vi "modbus slave new.vi"() -> ()   [LabVIEW 2016, in "MB SLAVE.lvlib"]
uses:
  MB SLAVE.lvlib
  <vilib>/NI/Modbus Library/Network Protocol/Network Slave/daemon status.ctl
  <vilib>/NI/Modbus Library/Network Protocol/Network Slave/TCP/Connection.ctl
  <vilib>/NI/Modbus Library/API/slave/Modbus Slave.lvclass
  <vilib>/NI/Modbus Library/API/Wrapper/Create TCP Slave.vi
  <vilib>/NI/Modbus Library/API/Wrapper/API Main.lvlib
  <vilib>/ptbypt/NI_PtbyPt.lvlib
  <vilib>/NI/Modbus Library/Network Protocol/Network Slave/Network Slave.lvclass
  <vilib>/NI/Modbus Library/Network Protocol/Network Slave/TCP/TCP Slave.lvclass
panel:
  out "MB引用":refnum<class "Modbus Slave.lvclass">
  out "读取采水泵阀":u16[](array[numeric])
  out "读取数采仪软件版本":u16[](array[numeric])
  in  "写入数据传输软件升级":u16[](array[numeric])
  in  "写入仪器固件":u16[](array[numeric])
  in  "写入系统信息":u16[](array[numeric])
  in  "写入系统版本信息":u16[](array[numeric])
  in  "写入仪器告警信息":u16[](array[numeric])
  in  "写入采配水关键参数":u16[](array[numeric])
  in  "写入校准点信息":u16[](array[numeric])
  in  "写入关键参数":u16[](array[numeric])
  in  "写入各参数测量间隔":u16[](array[numeric])
  out "读取各参数测量间隔":u16[](array[numeric])
  in  "写入试剂余量":u16[](array[numeric])
  out "TCP Connection List":T1[](array[typedef])
  out "TCP Connection Count":u32
  out "Daemon Status":T2
  out "读取关键参数":u16[](array[numeric])
  out "status":bool
  in  "写入系统仪器状态":u16[](array[numeric])
  out "读取反控命令":u16[](array[numeric])
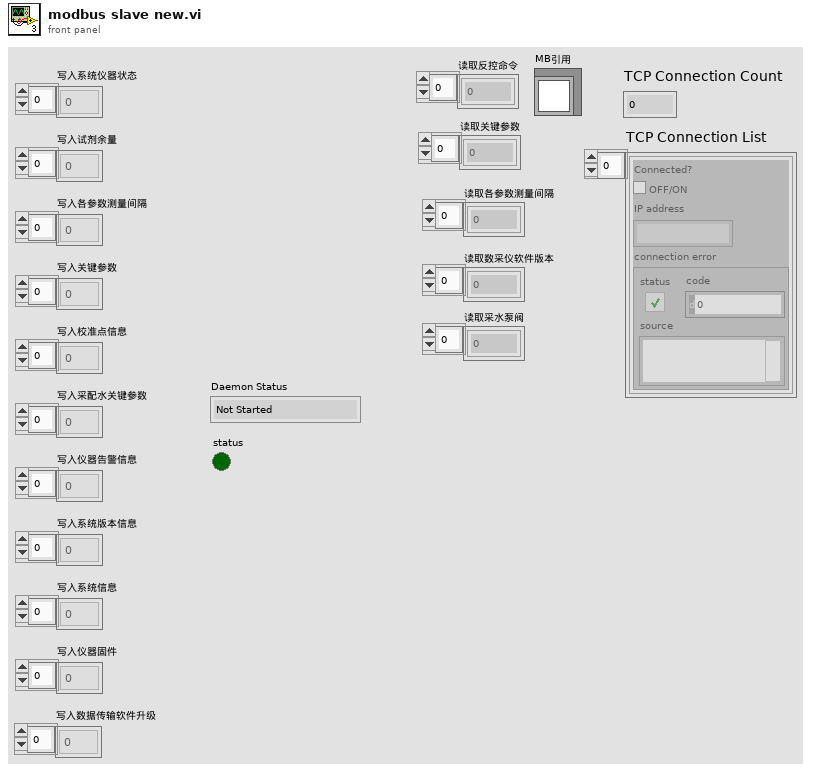
[diagram p1: front panel]
types:
  T1 = typedef "TCP Slave.lvclass/Connection.ctl" = cluster{"Connected?":bool, "IP address":string, "connection error":errorcluster}
  T2 = typedef "Network Slave.lvclass/daemon status.ctl" = enum16{"Not Started", "Running", "Error", "Stopped"}
  T3 = enum16{"", "CODMn", "PH", "氨氮", "总氮", "总磷", "CODCr", "电导率", "水温", "溶解氧", "浊度", "叶绿素", "藻密度", "ORP"}
  T4 = enum16{"i13001", "i13002", "i13003", "i13004", "i13005", "i13006", "i13007", "i13008", "i13009", "i13010", "i13011", "i13012", "i13013", "i13014", "i13015", "i13016", "i13017", "i13101", "i13102", "i13103", "i13104", "i13105", "i13106", "i13107", "i13108", "i13109", "i13110"}
  T5 = cluster{"status":bool, "代码":u16, "source":string}
  T6 = typedef "系统交互.ctl" = cluster{"运行模式":enum16{"维护模式", "常规模式", "应急模式", "质控模式", "性能测试"}, "运行间隔":i16, "流程运行中":bool, "自动运行启动参数":T7, "SYSTEM Interface.总磷总氮类型":enum16{"单模块", "总磷总氮二合一模块", "氨氮总磷二合一模块"}, "多参数运行间隔":i16, "配水时间":dbl, "沉淀时间":dbl, "清洗时间":dbl, "关键参数改变":bool, "温度告警":bool, "湿度告警":bool, "烟感告警":bool, "水浸告警":bool, "开门告警":bool, "SystemTask":enum16{"停机", "待机", "调试", "水样采集", "沉沙", "进样", "仪表测试分析", "反吹", "清洗", "除藻"}, "PumpState":enum16{"--", "只用泵1", "只用泵2", "双泵交替"}, "除藻选择":enum16{"不开除藻", "开除藻"}, "报警信息":enum16{"无报警", "断电报警", "采样管理欠压（源水泵故障）", "进样管路欠压（进样泵/增加泵故障）"}, "软件升级":bool, "固件升级":enum16{"无", "CODMn", "氨氮", "总磷", "总氮", "CODCr"}, "数据传输软件升级":bool, "数采仪软件版本":string}
  T7 = typedef "启动参数.ctl" = cluster{"氨氮":bool, "总磷":bool, "总氮":bool, "多参数":bool, "CODmn":bool, "CODCr":bool, "超标留样":bool}
  T8 = enum16{"停机", "待机", "调试", "水样采集", "沉沙", "进样", "仪表测试分析", "反吹", "清洗", "除藻"}
  T9 = enum16{"无报警", "断电报警", "采样管理欠压（源水泵故障）", "进样管路欠压（进样泵/增加泵故障）"}
  T10 = typedef "多参数交互.ctl" = cluster{"pH":bool, "DO":bool, "Turb":bool, "Cond":bool, "Temp":bool, "叶绿素a启用":bool, "蓝绿藻":bool, "藻密度":bool, "orp":bool}
  T11 = typedef "CODMn交互.ctl" = cluster{"COD浓度（mg/L)":dbl, "水样启动时间":timestamp, "加标回收启动时间":timestamp, "CODMn工作状态":enum16{"空闲", "水样测试", "标样核查", "零点核查", "跨度核查", "空白测试", "平行样测试", "加标回收", "空白校准", "标样校准", "初始化（清洗）"}, "多列列表框":i32, "平台试剂余量百分比":sgl, "关键参数":cluster{"测量量程":dbl, "测量精度":dbl, "测量间隔":dbl, "消解温度":dbl, "消解时长":dbl, "空白校准时间":timestamp, "曲线截距":dbl, "曲线斜率":dbl, "测量检出限":dbl, "测量信号值":dbl, "线性相关系数":dbl, "二次多项式系数":dbl, "标样校准时间":timestamp, "稀释倍数":dbl, "三项式系数":dbl, "空白标定系数":dbl, "量程系数":dbl, "F0/ORPA":dbl, "F1/ORPB":dbl, "F2/ORPK":dbl, "F3":dbl, "F4":dbl, "F5":dbl, "F6":dbl, "F7":dbl, "X0/滴定数":dbl, "量程":dbl}, "关键参数改变":bool, "校准信息":cluster{"低标液1浓度":dbl, "低标液1信号值":dbl, "低标液1启用":u16, "低标液2浓度":dbl, "低标液2信号值":dbl, "低标液2启用":u16, "低标液3浓度":dbl, "低标液3信号值":dbl, "低标液3启用":u16, "低标液4浓度":dbl, "低标液4信号值":dbl, "低标液4启用":u16, "低标液5浓度":dbl, "低标液5信号值":dbl, "低标液5启用":u16, "高标液1浓度":dbl, "高标液1信号值":dbl, "高标液1启用":u16, "高标液2浓度":dbl, "高标液2信号值":dbl, "高标液2启用":u16, "高标液3浓度":dbl, "高标液3信号值":dbl, "高标液3启用":u16, "高标液4浓度":dbl, "高标液4信号值":dbl, "高标液4启用":u16, "高标液5浓度":dbl, "高标液5信号值":dbl, "高标液5启用":u16, "低斜率":dbl, "低截距":dbl, "低二次多项式系数":dbl, "低线性相关系数":dbl, "高斜率":dbl, "高截距":dbl, "高二次多项式系数":dbl, "高线性相关系数":dbl}, "校准信息改变":bool, "固件版本号":string, "CODMn模块版本":T12, "协议":u16, "状态告警区":cluster{"系统时间":timestamp, "工作状态":u16, "测量模式":enum16{"待机", "连续模式", "周期模式", "定点模式", "受控模式", "手动模式"}, "告警代码":u16, "故障代码":u16, "日志代码":u16, "软件版本":u16, "F0":sgl, "F1":sgl, "F2":sgl, "F3":sgl, "T":sgl, "H":sgl, "id":u16, "flowid":u16, "量程":u16, "总磷控温温度1":sgl, "营养盐控温温度2":sgl, "ADC":sgl}, "标样核查标液浓度":dbl, "测量数据区":cluster{"空白数据时间":timestamp, "空白实测值":sgl, "标样数据时间":timestamp, "标样实测值":sgl}}
  T12 = typedef "CODMn模块版本.ctl" = enum16{"PLC版", "单片机版", "通用流路版本"}
  T13 = typedef "CODCr交互.ctl" = cluster{"状态告警区":cluster{"系统时间":timestamp, "工作状态":u16, "测量模式":enum16{"待机", "连续模式", "周期模式", "定点模式", "受控模式", "手动模式"}, "告警代码":u16, "故障代码":u16, "日志代码":u16, "软件版本":u16, "F0":sgl, "F1":sgl, "F2":sgl, "F3":sgl, "T":sgl, "H":sgl, "id":u16, "flowid":u16, "量程":u16, "总磷控温温度1":sgl, "营养盐控温温度2":sgl, "ADC":sgl}, "平台试剂余量百分比":sgl, "关键参数":cluster{"测量量程":dbl, "测量精度":dbl, "测量间隔":dbl, "消解温度":dbl, "消解时长":dbl, "空白校准时间":timestamp, "曲线截距":dbl, "曲线斜率":dbl, "测量检出限":dbl, "测量信号值":dbl, "线性相关系数":dbl, "二次多项式系数":dbl, "标样校准时间":timestamp, "稀释倍数":dbl, "三项式系数":dbl, "空白标定系数":dbl, "量程系数":dbl, "F0/ORPA":dbl, "F1/ORPB":dbl, "F2/ORPK":dbl, "F3":dbl, "F4":dbl, "F5":dbl, "F6":dbl, "F7":dbl, "X0/滴定数":dbl, "量程":dbl}, "关键参数改变":bool, "校准信息":cluster{"低标液1浓度":dbl, "低标液1信号值":dbl, "低标液1启用":u16, "低标液2浓度":dbl, "低标液2信号值":dbl, "低标液2启用":u16, "低标液3浓度":dbl, "低标液3信号值":dbl, "低标液3启用":u16, "低标液4浓度":dbl, "低标液4信号值":dbl, "低标液4启用":u16, "低标液5浓度":dbl, "低标液5信号值":dbl, "低标液5启用":u16, "高标液1浓度":dbl, "高标液1信号值":dbl, "高标液1启用":u16, "高标液2浓度":dbl, "高标液2信号值":dbl, "高标液2启用":u16, "高标液3浓度":dbl, "高标液3信号值":dbl, "高标液3启用":u16, "高标液4浓度":dbl, "高标液4信号值":dbl, "高标液4启用":u16, "高标液5浓度":dbl, "高标液5信号值":dbl, "高标液5启用":u16, "低斜率":dbl, "低截距":dbl, "低二次多项式系数":dbl, "低线性相关系数":dbl, "高斜率":dbl, "高截距":dbl, "高二次多项式系数":dbl, "高线性相关系数":dbl}, "校准信息改变":bool, "固件版本号":string}
  T14 = typedef "氨氮交互.ctl" = cluster{"状态告警区":cluster{"系统时间":timestamp, "工作状态":u16, "测量模式":enum16{"待机", "连续模式", "周期模式", "定点模式", "受控模式", "手动模式"}, "告警代码":u16, "故障代码":u16, "日志代码":u16, "软件版本":u16, "F0":sgl, "F1":sgl, "F2":sgl, "F3":sgl, "T":sgl, "H":sgl, "id":u16, "flowid":u16, "量程":u16, "总磷控温温度1":sgl, "营养盐控温温度2":sgl, "ADC":sgl}, "平台试剂余量百分比":sgl, "关键参数":cluster{"测量量程":dbl, "测量精度":dbl, "测量间隔":dbl, "消解温度":dbl, "消解时长":dbl, "空白校准时间":timestamp, "曲线截距":dbl, "曲线斜率":dbl, "测量检出限":dbl, "测量信号值":dbl, "线性相关系数":dbl, "二次多项式系数":dbl, "标样校准时间":timestamp, "稀释倍数":dbl, "三项式系数":dbl, "空白标定系数":dbl, "量程系数":dbl, "F0/ORPA":dbl, "F1/ORPB":dbl, "F2/ORPK":dbl, "F3":dbl, "F4":dbl, "F5":dbl, "F6":dbl, "F7":dbl, "X0/滴定数":dbl, "量程":dbl}, "关键参数改变":bool, "校准信息":cluster{"低标液1浓度":dbl, "低标液1信号值":dbl, "低标液1启用":u16, "低标液2浓度":dbl, "低标液2信号值":dbl, "低标液2启用":u16, "低标液3浓度":dbl, "低标液3信号值":dbl, "低标液3启用":u16, "低标液4浓度":dbl, "低标液4信号值":dbl, "低标液4启用":u16, "低标液5浓度":dbl, "低标液5信号值":dbl, "低标液5启用":u16, "高标液1浓度":dbl, "高标液1信号值":dbl, "高标液1启用":u16, "高标液2浓度":dbl, "高标液2信号值":dbl, "高标液2启用":u16, "高标液3浓度":dbl, "高标液3信号值":dbl, "高标液3启用":u16, "高标液4浓度":dbl, "高标液4信号值":dbl, "高标液4启用":u16, "高标液5浓度":dbl, "高标液5信号值":dbl, "高标液5启用":u16, "低斜率":dbl, "低截距":dbl, "低二次多项式系数":dbl, "低线性相关系数":dbl, "高斜率":dbl, "高截距":dbl, "高二次多项式系数":dbl, "高线性相关系数":dbl}, "校准信息改变":bool, "固件版本号":string}
  T15 = typedef "总磷交互.ctl" = cluster{"状态告警区":cluster{"系统时间":timestamp, "工作状态":u16, "测量模式":enum16{"待机", "连续模式", "周期模式", "定点模式", "受控模式", "手动模式"}, "告警代码":u16, "故障代码":u16, "日志代码":u16, "软件版本":u16, "F0":sgl, "F1":sgl, "F2":sgl, "F3":sgl, "T":sgl, "H":sgl, "id":u16, "flowid":u16, "量程":u16, "总磷控温温度1":sgl, "营养盐控温温度2":sgl, "ADC":sgl}, "平台试剂余量百分比":sgl, "关键参数":cluster{"测量量程":dbl, "测量精度":dbl, "测量间隔":dbl, "消解温度":dbl, "消解时长":dbl, "空白校准时间":timestamp, "曲线截距":dbl, "曲线斜率":dbl, "测量检出限":dbl, "测量信号值":dbl, "线性相关系数":dbl, "二次多项式系数":dbl, "标样校准时间":timestamp, "稀释倍数":dbl, "三项式系数":dbl, "空白标定系数":dbl, "量程系数":dbl, "F0/ORPA":dbl, "F1/ORPB":dbl, "F2/ORPK":dbl, "F3":dbl, "F4":dbl, "F5":dbl, "F6":dbl, "F7":dbl, "X0/滴定数":dbl, "量程":dbl}, "关键参数改变":bool, "校准信息":cluster{"低标液1浓度":dbl, "低标液1信号值":dbl, "低标液1启用":u16, "低标液2浓度":dbl, "低标液2信号值":dbl, "低标液2启用":u16, "低标液3浓度":dbl, "低标液3信号值":dbl, "低标液3启用":u16, "低标液4浓度":dbl, "低标液4信号值":dbl, "低标液4启用":u16, "低标液5浓度":dbl, "低标液5信号值":dbl, "低标液5启用":u16, "高标液1浓度":dbl, "高标液1信号值":dbl, "高标液1启用":u16, "高标液2浓度":dbl, "高标液2信号值":dbl, "高标液2启用":u16, "高标液3浓度":dbl, "高标液3信号值":dbl, "高标液3启用":u16, "高标液4浓度":dbl, "高标液4信号值":dbl, "高标液4启用":u16, "高标液5浓度":dbl, "高标液5信号值":dbl, "高标液5启用":u16, "低斜率":dbl, "低截距":dbl, "低二次多项式系数":dbl, "低线性相关系数":dbl, "高斜率":dbl, "高截距":dbl, "高二次多项式系数":dbl, "高线性相关系数":dbl}, "校准信息改变":bool, "固件版本号":string}
  T16 = typedef "总氮交互.ctl" = cluster{"状态告警区":cluster{"系统时间":timestamp, "工作状态":u16, "测量模式":enum16{"待机", "连续模式", "周期模式", "定点模式", "受控模式", "手动模式"}, "告警代码":u16, "故障代码":u16, "日志代码":u16, "软件版本":u16, "F0":sgl, "F1":sgl, "F2":sgl, "F3":sgl, "T":sgl, "H":sgl, "id":u16, "flowid":u16, "量程":u16, "总磷控温温度1":sgl, "营养盐控温温度2":sgl, "ADC":sgl}, "平台试剂余量百分比":sgl, "关键参数":cluster{"测量量程":dbl, "测量精度":dbl, "测量间隔":dbl, "消解温度":dbl, "消解时长":dbl, "空白校准时间":timestamp, "曲线截距":dbl, "曲线斜率":dbl, "测量检出限":dbl, "测量信号值":dbl, "线性相关系数":dbl, "二次多项式系数":dbl, "标样校准时间":timestamp, "稀释倍数":dbl, "三项式系数":dbl, "空白标定系数":dbl, "量程系数":dbl, "F0/ORPA":dbl, "F1/ORPB":dbl, "F2/ORPK":dbl, "F3":dbl, "F4":dbl, "F5":dbl, "F6":dbl, "F7":dbl, "X0/滴定数":dbl, "量程":dbl}, "关键参数改变":bool, "校准信息":cluster{"低标液1浓度":dbl, "低标液1信号值":dbl, "低标液1启用":u16, "低标液2浓度":dbl, "低标液2信号值":dbl, "低标液2启用":u16, "低标液3浓度":dbl, "低标液3信号值":dbl, "低标液3启用":u16, "低标液4浓度":dbl, "低标液4信号值":dbl, "低标液4启用":u16, "低标液5浓度":dbl, "低标液5信号值":dbl, "低标液5启用":u16, "高标液1浓度":dbl, "高标液1信号值":dbl, "高标液1启用":u16, "高标液2浓度":dbl, "高标液2信号值":dbl, "高标液2启用":u16, "高标液3浓度":dbl, "高标液3信号值":dbl, "高标液3启用":u16, "高标液4浓度":dbl, "高标液4信号值":dbl, "高标液4启用":u16, "高标液5浓度":dbl, "高标液5信号值":dbl, "高标液5启用":u16, "低斜率":dbl, "低截距":dbl, "低二次多项式系数":dbl, "低线性相关系数":dbl, "高斜率":dbl, "高截距":dbl, "高二次多项式系数":dbl, "高线性相关系数":dbl}, "校准信息改变":bool, "固件版本号":string}
  T17 = cluster{"测量量程":dbl, "测量精度":dbl, "测量间隔":dbl, "消解温度":dbl, "消解时长":dbl, "空白校准时间":timestamp, "曲线截距":dbl, "曲线斜率":dbl, "测量检出限":dbl, "测量信号值":dbl, "线性相关系数":dbl, "二次多项式系数":dbl, "标样校准时间":timestamp, "稀释倍数":dbl, "三项式系数":dbl, "空白标定系数":dbl, "量程系数":dbl, "F0/ORPA":dbl, "F1/ORPB":dbl, "F2/ORPK":dbl, "F3":dbl, "F4":dbl, "F5":dbl, "F6":dbl, "F7":dbl, "X0/滴定数":dbl, "量程":dbl}
  T18 = cluster{"低标液1浓度":dbl, "低标液1信号值":dbl, "低标液1启用":u16, "低标液2浓度":dbl, "低标液2信号值":dbl, "低标液2启用":u16, "低标液3浓度":dbl, "低标液3信号值":dbl, "低标液3启用":u16, "低标液4浓度":dbl, "低标液4信号值":dbl, "低标液4启用":u16, "低标液5浓度":dbl, "低标液5信号值":dbl, "低标液5启用":u16, "高标液1浓度":dbl, "高标液1信号值":dbl, "高标液1启用":u16, "高标液2浓度":dbl, "高标液2信号值":dbl, "高标液2启用":u16, "高标液3浓度":dbl, "高标液3信号值":dbl, "高标液3启用":u16, "高标液4浓度":dbl, "高标液4信号值":dbl, "高标液4启用":u16, "高标液5浓度":dbl, "高标液5信号值":dbl, "高标液5启用":u16, "低斜率":dbl, "低截距":dbl, "低二次多项式系数":dbl, "低线性相关系数":dbl, "高斜率":dbl, "高截距":dbl, "高二次多项式系数":dbl, "高线性相关系数":dbl}
  T19 = enum16{"空闲", "水样测试", "标样核查", "零点核查", "跨度核查", "空白测试", "平行样测试", "加标回收", "空白校准", "标样校准", "初始化（清洗）"}
  T20 = typedef "超标留样交互.ctl" = cluster{"当前瓶号":u16}
  T21 = cluster{"测量量程":dbl, "测量精度":dbl, "测量间隔":dbl, "消解温度":dbl, "消解时长":dbl, "空白校准时间":timestamp, "曲线截距":dbl, "曲线斜率":dbl, "测量检出限":dbl, "测量信号值":dbl, "线性相关系数":dbl, "二次多项式系数":dbl, "标样校准时间":timestamp, "稀释倍数":dbl, "三项式系数":dbl, "空白标定系数":dbl, "量程系数":dbl, "F0/ORPA":dbl, "F1/ORPB":dbl, "F2/ORPK":dbl, "F3":dbl, "F4":dbl, "F5":dbl, "F6":dbl, "F7":dbl, "X0/滴定数":dbl, "量程":dbl}[]
  T22 = cluster{"低标液1浓度":dbl, "低标液1信号值":dbl, "低标液1启用":u16, "低标液2浓度":dbl, "低标液2信号值":dbl, "低标液2启用":u16, "低标液3浓度":dbl, "低标液3信号值":dbl, "低标液3启用":u16, "低标液4浓度":dbl, "低标液4信号值":dbl, "低标液4启用":u16, "低标液5浓度":dbl, "低标液5信号值":dbl, "低标液5启用":u16, "高标液1浓度":dbl, "高标液1信号值":dbl, "高标液1启用":u16, "高标液2浓度":dbl, "高标液2信号值":dbl, "高标液2启用":u16, "高标液3浓度":dbl, "高标液3信号值":dbl, "高标液3启用":u16, "高标液4浓度":dbl, "高标液4信号值":dbl, "高标液4启用":u16, "高标液5浓度":dbl, "高标液5信号值":dbl, "高标液5启用":u16, "低斜率":dbl, "低截距":dbl, "低二次多项式系数":dbl, "低线性相关系数":dbl, "高斜率":dbl, "高截距":dbl, "高二次多项式系数":dbl, "高线性相关系数":dbl}[]
  T23 = typedef "MB SLAVE.lvlib/启动命令类型.ctl" = enum16{"启动整机", "停止整机", "标样核查", "加标回收", "平行样测试", "零点核查", "跨度核查", "校零", "校标", "启动系统全面清洗", "水样测试", "启动采水泵阀", "仪表校准", "仪表重启"}
  T24 = typedef "采配水交互.ctl" = cluster{"测试模式":enum16{"清洗", "开泵X", "开阀X", "关泵X", "关阀X"}, "值":u16}
  T25 = cluster{"时间标识":timestamp, "设备":string, "日志信息":string, "流程参数":string}
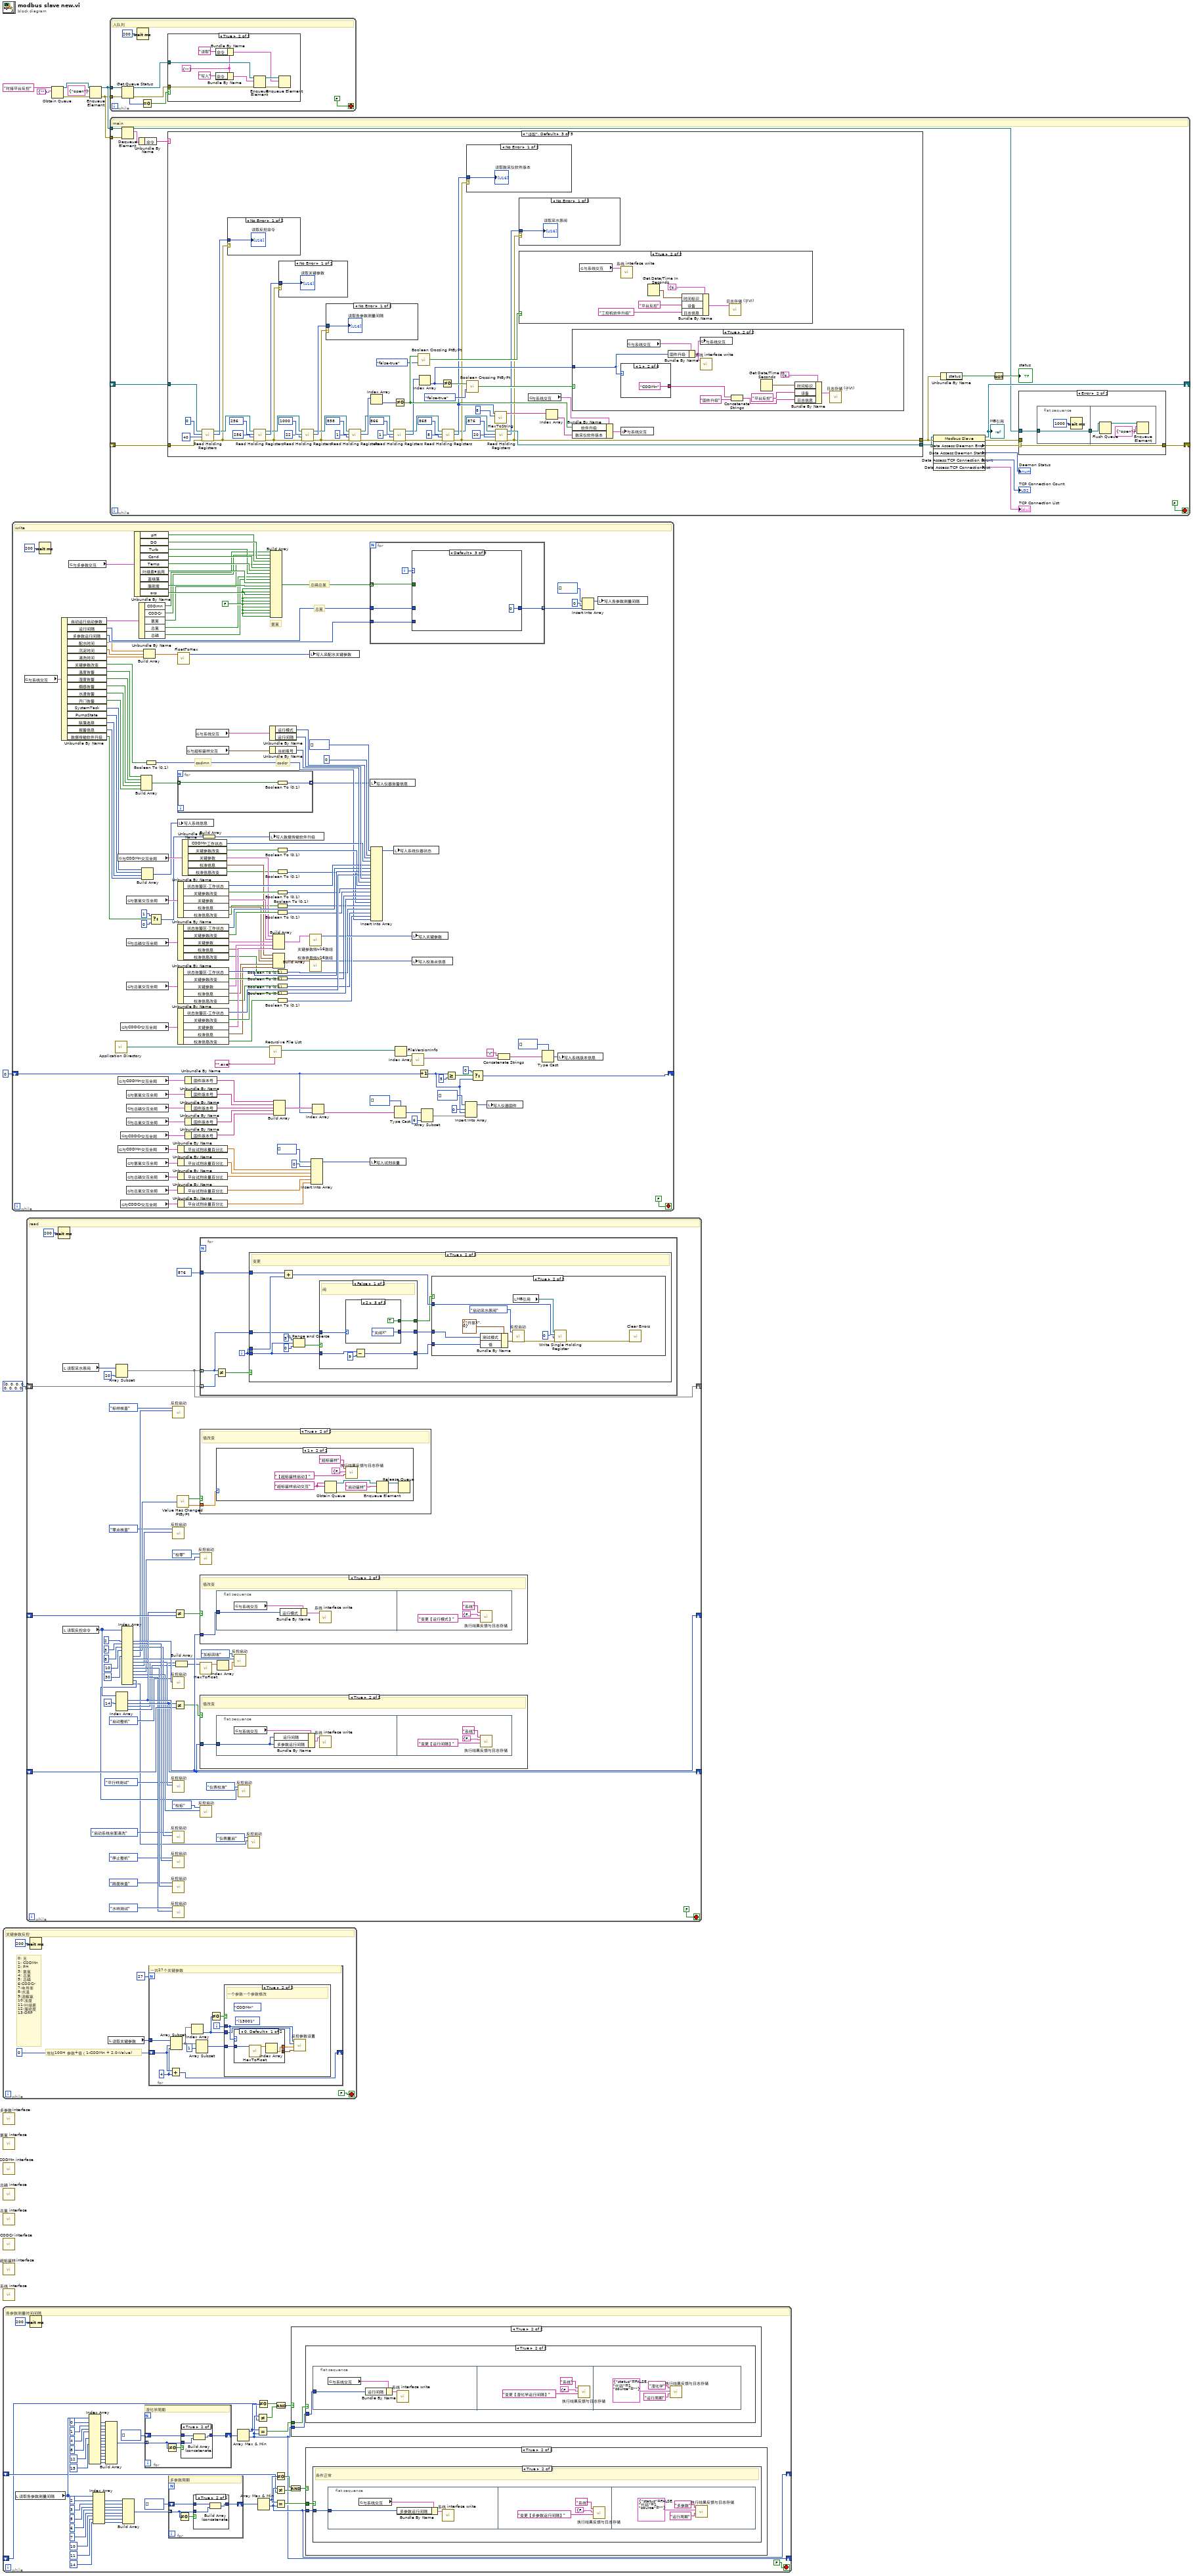
[diagram p0: block diagram]
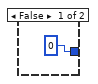
[diagram p3: hidden frame]
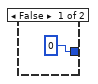
[diagram p5: hidden frame]
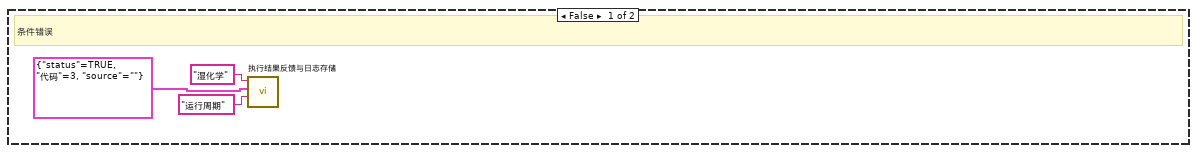
[diagram p7: hidden frame]
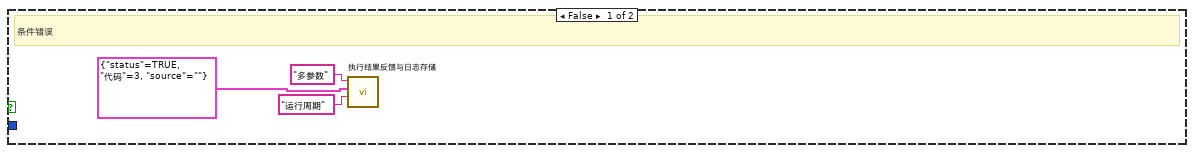
[diagram p9: hidden frame]
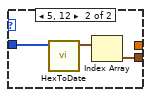
[diagram p13: hidden frame]
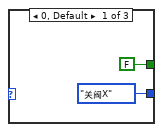
[diagram p16: hidden frame]
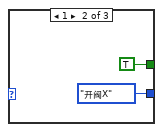
[diagram p17: hidden frame]
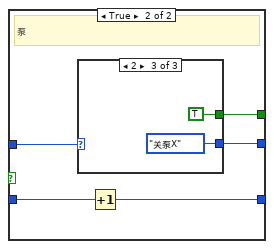
[diagram p18: hidden frame]
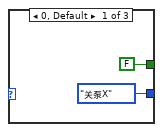
[diagram p19: hidden frame]
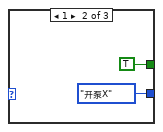
[diagram p20: hidden frame]
diagram:
  n1 = while {
    stop <- FALSE stop-if-true
    # "地址100H 参数+值（1-CODMn + 2.0-Value)"
    # "0: 无\n1: CODMn\n2: PH\n3: 氨氮\n4: 总氮\n5: 总磷\n6:CODCr\n7:电导率\n8:水温\n9:溶解氧\n10:浊度\n11:叶绿素\n12:藻密度\n13:ORP"
    # "关键参数反控"
    n2 = Wait (ms)(milliseconds to wait=u32 200 ("等待时间（毫秒）")) -> ()  [unwired: 1 out]
    n3 = local read "读取关键参数"() -> (w12:u16[])
    n4 = for {
      N: 27 -> [_]
      tunnel: w12 -> [w24]
      shift-right: [w15] -> _
      shift-left: 0 ("索引") -> [w17]
      i -> [w20]
      w16 = 4 ("长度")
      # "一共27个关键参数"
      n5 = Add(x=w17, y=w16) -> (x+y=w15:i32)
      n6 = Array Subset(array=w24, index=w17, length=w16) -> (w23:u16[])
      n7 = Index Array(array=w23) -> (element=w19:u16)  [unwired: 1 in]
      n8 = Array Subset(array=w23, index=1 ("索引")) -> (w21:u16[])  [unwired: 1 in]
      n9 = Not Equal To 0?(x=w19) -> (x != 0?=w18:bool)
      n10 = case shown="True" w18 {
        tunnel: w21 -> [_ w29]
        tunnel: w20 -> [_ w28]
        tunnel: w19 -> [_ w27]
        frame False {
        }
        frame True {
          (unwired) T3."CODMn"
          (unwired) T4."i13001" ("设置类型")
          # "一个参数一个参数修改"
          n11 = case shown="0, Default" w28 {
            tunnel: w29 -> [w31 w34]
            tunnel: [_ w35] -> w25
            tunnel: [w32 _] -> w26
            frame 0, Default {
              n12 = call "HexToFloat.vi"("数组"=w31) -> ("FLOAT"=w30:sgl[])  [unwired: 10 in]
              n13 = Index Array(array=w30) -> (element=w32:sgl)  [unwired: 1 in]
            }
            frame 5, 12 {
              n14 = call "HexToDate.vi"("数组"=w34) -> ("DATE"=w33:timestamp[])  [unwired: 10 in]
              n15 = Index Array(array=w33) -> (element=w35:timestamp)  [unwired: 1 in]
            }
          }
          n16 = call "反控参数设置.vi"("value time"=w25, "value float"=w26, "设置参数"=w27, "设置类型"=w28) -> ()  [unwired: 8 in]
        }
      }
    }
  }
  n17 = call "多参数 interface.vi"() -> ()  [unwired: 12 in]
  n18 = call "氨氮 interface.vi"() -> ()  [unwired: 12 in]
  n19 = call "CODMn interface.vi"() -> ()  [unwired: 12 in]
  n20 = call "总磷 interface.vi"() -> ()  [unwired: 12 in]
  n21 = call "总氮 interface.vi"() -> ()  [unwired: 12 in]
  n22 = call "CODCr interface.vi"() -> ()  [unwired: 12 in]
  n23 = call "超标留样 interface.vi"() -> ()  [unwired: 12 in]
  n24 = call "系统 interface.vi"() -> ()  [unwired: 12 in]
  n25 = while {
    shift-right: [w47] -> _
    shift-left: _ -> [w46]
    shift-right: [w40] -> _
    shift-left: _ -> [w39]
    stop <- FALSE stop-if-true
    # "各参数测量时间间隔"
    n26 = local read "读取各参数测量间隔"() -> (w88:u16[])
    n27 = Wait (ms)(milliseconds to wait=u32 200 ("等待时间（毫秒）")) -> ()  [unwired: 1 out]
    n28 = Index Array(array=w88, index #1=0 ("索引"), index #2=1 ("索引"), index #3=4 ("索引"), index #4=8 ("索引"), index #6=12 ("索引"), index #8=15 ("索引")) -> (element #1=w69:u16, element #2=w68:u16, element #3=w67:u16, element #4=w66:u16, element #5=w65:u16, element #6=w64:u16, element #7=w63:u16, element #8=w62:u16, element #9=w61:u16, element #10=w60:u16, element #11=w59:u16, element #12=w58:u16, element #13=w57:u16, element #14=w56:u16)  [unwired: 8 in]
    n29 = Index Array(array=w88, index #1=2 ("索引"), index #2=3 ("索引"), index #3=5 ("索引"), index #4=6 ("索引"), index #5=7 ("索引"), index #6=10 ("索引"), index #7=11 ("索引"), index #8=14 ("索引")) -> (element #1=w77:u16, element #2=w76:u16, element #3=w75:u16, element #4=w74:u16, element #5=w73:u16, element #6=w72:u16, element #7=w71:u16, element #8=w70:u16)
    n30 = Build Array(w69, w68, w67, w66, w65, w64, w63, w62, w61, w60, w59, w58, w57, w56) -> (w51:u16[])
    n31 = Build Array(w77, w76, w75, w74, w73, w72, w71, w70) -> (w55:u16[])
    n32 = for {
      shift-right: [w126] -> w50
      shift-left: u16[] [] ("添加的数组") -> [w127]
      tunnel: w51 -> [w125] mode=indexing
      # "湿化学周期"
      n33 = Not Equal To 0?(x=w125) -> (x != 0?=w128:bool)
      n34 = case shown="True" w128 {
        tunnel: w127 -> [w129 w132]
        tunnel: w125 -> [_ w131]
        tunnel: [w129 w130] -> w126
        frame False {
        }
        frame True {
          n35 = Build Array (concatenate)(w132, w131) -> (w130:u16[])
        }
      }
    }
    n36 = for {
      tunnel: w55 -> [w135] mode=indexing
      shift-right: [w133] -> w53
      shift-left: u16[] [] ("添加的数组") -> [w136]
      # "多参数周期"
      n37 = Not Equal To 0?(x=w135) -> (x != 0?=w134:bool)
      n38 = case shown="True" w134 {
        tunnel: w136 -> [w137 w140]
        tunnel: w135 -> [_ w139]
        tunnel: [w137 w138] -> w133
        frame False {
        }
        frame True {
          n39 = Build Array (concatenate)(w140, w139) -> (w138:u16[])
        }
      }
    }
    n40 = Array Max & Min(array=w50) -> (max value=w49:u16, min value=w40:u16)  [unwired: 2 out]
    n41 = Not Equal?(x=w40, y=w39) -> (x != y?=w38:bool)
    n42 = Equal?(x=w49, y=w40) -> (x = y?=w36:bool)
    n43 = Not Equal To 0?(x=w49) -> (x != 0?=w41:bool)
    n44 = Array Max & Min(array=w53) -> (max value=w48:u16, min value=w47:u16)  [unwired: 2 out]
    n45 = Not Equal To 0?(x=w48) -> (x != 0?=w45:bool)
    n46 = Not Equal?(x=w47, y=w46) -> (x != y?=w44:bool)
    n47 = Equal?(x=w48, y=w47) -> (x = y?=w42:bool)
    n48 = And(x=w41, y=w38) -> (x .and. y?=w37:bool)
    n49 = And(x=w45, y=w44) -> (x .and. y?=w43:bool)
    n50 = case shown="True" w37 {
      tunnel: w40 -> [_ w96]
      tunnel: w36 -> [_ w95]
      frame False {
        # "值未改变"
      }
      frame True {
        n51 = case shown="True" w95 {
          tunnel: w96 -> [_ w100]
          frame False {
            # "条件错误"
            n52 = call "执行结果反馈与日志存储.vi"("日志信息"="运行周期", "error out"=T5 {"status"=TRUE, "代码"=3, "source"=""}, "设备"="湿化学") -> ()  [unwired: 9 in]
          }
          frame True {
            n53 = flat-sequence {
              tunnel: w100 -> [w102]
              frame #0 {
                n54 = global read "modbus slave全局.vi" "与系统交互"() -> (w103:T6)
                n55 = Bundle By Name(cluster=w103, "运行间隔"=w102) -> (w101:T6)
                n56 = call "系统 interface write.vi"("与系统交互"=w101) -> ()  [unwired: 11 in]
              }
              frame #1 {
                n57 = call "执行结果反馈与日志存储.vi"("日志信息"="变更【湿化学运行间隔】", "error out"=T5 {"status"=FALSE, "代码"=1, "source"=""}, "设备"="系统") -> ()  [unwired: 9 in]
              }
              frame #2 {
                n58 = call "执行结果反馈与日志存储.vi"("日志信息"="运行周期", "error out"=T5 {"status"=FALSE, "代码"=1, "source"=""}, "设备"="湿化学") -> ()  [unwired: 9 in]
              }
            }
          }
        }
      }
    }
    n59 = case shown="True" w43 {
      tunnel: w47 -> [_ w111]
      tunnel: w42 -> [_ w110]
      frame False {
        # "值未改变"
      }
      frame True {
        n60 = case shown="True" w110 {
          tunnel: w111 -> [_ w115]
          frame False {
            # "条件错误"
            n61 = call "执行结果反馈与日志存储.vi"("日志信息"="运行周期", "error out"=T5 {"status"=TRUE, "代码"=3, "source"=""}, "设备"="多参数") -> ()  [unwired: 9 in]
          }
          frame True {
            # "条件正常"
            n62 = flat-sequence {
              tunnel: w115 -> [w117]
              frame #0 {
                n63 = global read "modbus slave全局.vi" "与系统交互"() -> (w118:T6)
                n64 = Bundle By Name(cluster=w118, "多参数运行间隔"=w117) -> (w116:T6)
                n65 = call "系统 interface write.vi"("与系统交互"=w116) -> ()  [unwired: 11 in]
              }
              frame #1 {
                n66 = call "执行结果反馈与日志存储.vi"("日志信息"="变更【多参数运行间隔】", "error out"=T5 {"status"=FALSE, "代码"=1, "source"=""}, "设备"="系统") -> ()  [unwired: 9 in]
              }
              frame #2 {
                n67 = call "执行结果反馈与日志存储.vi"("日志信息"="运行周期", "error out"=T5 {"status"=FALSE, "代码"=1, "source"=""}, "设备"="多参数") -> ()  [unwired: 9 in]
              }
            }
          }
        }
      }
    }
  }
  n68 = while {
    shift-right: [w152] -> _
    shift-left: u16 0 ("索引") -> [w156]
    stop <- FALSE stop-if-true
    w243 = FALSE ("元素")
    # "总磷总氮"
    # "总氮"
    # "氨氮"
    # "codcr"
    # "codmn"
    # "write"
    n69 = global read "modbus slave全局.vi" "与系统交互"() -> (w256:T6)
    n70 = Wait (ms)(milliseconds to wait=u32 200 ("等待时间（毫秒）")) -> ()  [unwired: 1 out]
    n71 = Unbundle By Name(w256) -> ("自动运行启动参数"=w199:T7, "运行间隔"=w241:i16, "多参数运行间隔"=w240:i16, "配水时间"=w198:dbl, "沉淀时间"=w197:dbl, "清洗时间"=w196:dbl, "关键参数改变"=w193:bool, "温度告警"=w191:bool, "湿度告警"=w190:bool, "烟感告警"=w189:bool, "水浸告警"=w188:bool, "开门告警"=w187:bool, "SystemTask"=w175:T8, "PumpState"=w174:enum16{"--", "只用泵1", "只用泵2", "双泵交替"}, "除藻选择"=w173:enum16{"不开除藻", "开除藻"}, "报警信息"=w172:T9, "数据传输软件升级"=w143:bool)
    n72 = global read "modbus slave全局.vi" "与多参数交互"() -> (w255:T10)
    n73 = call <vilib>:"Application Directory.vi"() -> ("Application Directory"=w183:path)
    n74 = global read "modbus slave全局.vi" "与CODMn交互全局"() -> (w274:T11)
    n75 = global read "modbus slave全局.vi" "与CODMn交互全局"() -> (w167:T11)
    n76 = global read "modbus slave全局.vi" "与CODMn交互全局"() -> (w266:T11)
    n77 = global read "modbus slave全局.vi" "与CODCr交互全局"() -> (w282:T13)
    n78 = global read "modbus slave全局.vi" "与CODCr交互全局"() -> (w166:T13)
    n79 = global read "modbus slave全局.vi" "与CODCr交互全局"() -> (w262:T13)
    n80 = global read "modbus slave全局.vi" "与氨氮交互全局"() -> (w276:T14)
    n81 = global read "modbus slave全局.vi" "与总磷交互全局"() -> (w278:T15)
    n82 = global read "modbus slave全局.vi" "与总氮交互全局"() -> (w280:T16)
    n83 = global read "modbus slave全局.vi" "与氨氮交互全局"() -> (w163:T14)
    n84 = global read "modbus slave全局.vi" "与总磷交互全局"() -> (w164:T15)
    n85 = global read "modbus slave全局.vi" "与总氮交互全局"() -> (w165:T16)
    n86 = global read "modbus slave全局.vi" "与氨氮交互全局"() -> (w265:T14)
    n87 = global read "modbus slave全局.vi" "与总磷交互全局"() -> (w264:T15)
    n88 = global read "modbus slave全局.vi" "与总氮交互全局"() -> (w263:T16)
    n89 = Unbundle By Name(w255) -> ("pH"=w250:bool, "DO"=w251:bool, "Turb"=w247:bool, "Cond"=w249:bool, "Temp"=w248:bool, "叶绿素a启用"=w246:bool, "藻密度"=w245:bool, "orp"=w244:bool)  [unwired: 1 out]
    n90 = Unbundle By Name(w199) -> ("CODmn"=w204:bool, "CODCr"=w203:bool, "氨氮"=w202:bool, "总氮"=w201:bool, "总磷"=w200:bool)
    n91 = Build Array(w191, w190, w189, w188, w187) -> (w186:bool[])
    n92 = Build Array(w175, w174, w173, w172) -> (w171:u16[])
    n93 = Build Array(w198, w197, w196) -> (w195:dbl[])
    n94 = Boolean To (0,1)(Boolean=w193) -> (0, 1=w192:i16)
    n95 = Select(t=u16 1 ("Register"), s=w143, f=u16 0) -> (s? t:f=w142:u16)
    n96 = call "FloatToHex.vi"("FLOAT"=w195) -> ("交织的数组"=w194:u16[])  [unwired: 10 in]
    n97 = for {
      tunnel: w186 -> [w291] mode=indexing
      tunnel: [w290] -> w185 mode=indexing
      n98 = Boolean To (0,1)(Boolean=w291) -> (0, 1=w290:i16)
    }
    n99 = local write "写入系统信息"(w171) -> ()
    n100 = Unbundle By Name(w276) -> ("状态告警区.工作状态"=w277:u16, "关键参数改变"=w232:bool, "关键参数"=w227:T17, "校准信息"=w220:T18, "校准信息改变"=w214:bool)
    n101 = Unbundle By Name(w278) -> ("状态告警区.工作状态"=w279:u16, "关键参数改变"=w231:bool, "关键参数"=w226:T17, "校准信息"=w219:T18, "校准信息改变"=w212:bool)
    n102 = Unbundle By Name(w280) -> ("状态告警区.工作状态"=w281:u16, "关键参数改变"=w230:bool, "关键参数"=w225:T17, "校准信息"=w218:T18, "校准信息改变"=w210:bool)
    n103 = Unbundle By Name(w282) -> ("状态告警区.工作状态"=w283:u16, "关键参数改变"=w229:bool, "关键参数"=w224:T17, "校准信息"=w217:T18, "校准信息改变"=w208:bool)
    n104 = Unbundle By Name(w266) -> ("平台试剂余量百分比"=w261:sgl)
    n105 = Unbundle By Name(w265) -> ("平台试剂余量百分比"=w260:sgl)
    n106 = Unbundle By Name(w264) -> ("平台试剂余量百分比"=w259:sgl)
    n107 = Unbundle By Name(w263) -> ("平台试剂余量百分比"=w258:sgl)
    n108 = Unbundle By Name(w262) -> ("平台试剂余量百分比"=w257:sgl)
    n109 = Unbundle By Name(w274) -> ("CODMn工作状态"=w275:T19, "关键参数改变"=w233:bool, "关键参数"=w228:T17, "校准信息"=w221:T18, "校准信息改变"=w216:bool)
    n110 = Unbundle By Name(w167) -> ("固件版本号"=w162:string)
    n111 = Unbundle By Name(w163) -> ("固件版本号"=w161:string)
    n112 = Unbundle By Name(w164) -> ("固件版本号"=w160:string)
    n113 = Unbundle By Name(w165) -> ("固件版本号"=w159:string)
    n114 = Unbundle By Name(w166) -> ("固件版本号"=w158:string)
    n115 = global read "modbus slave全局.vi" "与超标留样交互"() -> (w287:T20)
    n116 = global read "modbus slave全局.vi" "与系统交互"() -> (w284:T6)
    n117 = Build Array(w142) -> (w141:u16[])
    n118 = Unbundle By Name(w284) -> ("运行模式"=w285:enum16{"维护模式", "常规模式", "应急模式", "质控模式", "性能测试"}, "运行间隔"=w286:i16)
    n119 = Unbundle By Name(w287) -> ("当前瓶号"=w288:u16)
    n120 = local write "写入数据传输软件升级"(w141) -> ()
    n121 = call <vilib>:"Recursive File List.vi"("pattern"="*.exe", "Folder Path"=w183) -> ("All Files in Dir"=w181:path[])  [unwired: 5 in, 4 out]
    n122 = Build Array(w204, w203, w251, w250, w202, w249, w248, w247, w201, w200, w246, w245, w243, w243, w244, w243, w243, w243, w243, w243, w243, w243) -> (w242:bool[])
    n123 = Build Array(w228, w227, w226, w225, w224) -> (w223:T21)
    n124 = Build Array(w221, w220, w219, w218, w217) -> (w206:T22)
    n125 = Build Array(w162, w161, w160, w159, w158) -> (w157:string[])
    n126 = Boolean To (0,1)(Boolean=w233) -> (0, 1=w238:i16)
    n127 = Boolean To (0,1)(Boolean=w216) -> (0, 1=w215:i16)
    n128 = Boolean To (0,1)(Boolean=w232) -> (0, 1=w237:i16)
    n129 = Boolean To (0,1)(Boolean=w214) -> (0, 1=w213:i16)
    n130 = Boolean To (0,1)(Boolean=w231) -> (0, 1=w236:i16)
    n131 = Boolean To (0,1)(Boolean=w212) -> (0, 1=w211:i16)
    n132 = Boolean To (0,1)(Boolean=w230) -> (0, 1=w235:i16)
    n133 = Boolean To (0,1)(Boolean=w210) -> (0, 1=w209:i16)
    n134 = Boolean To (0,1)(Boolean=w229) -> (0, 1=w234:i16)
    n135 = Boolean To (0,1)(Boolean=w208) -> (0, 1=w207:i16)
    n136 = local write "写入采配水关键参数"(w194) -> ()
    n137 = call "关键参数转u16数组.vi"("关键参数"=w223) -> ("添加的数组"=w222:u16[])  [unwired: 10 in]
    n138 = call "校准信息转u16数组.vi"("关键参数"=w206) -> ("添加的数组"=w205:u16[])  [unwired: 10 in]
    n139 = Insert Into Array(array=u16[] [] ("values to write"), index=0 ("索引"), new element #1=w261, new element #2=w260, new element #3=w259, new element #4=w258, new element #5=w257) -> (w269:u16[])
    n140 = Index Array(array=w157, index=w156) -> (element=w155:string)
    n141 = for {
      tunnel: w242 -> [w296] mode=indexing
      tunnel: w241 -> [w293]
      tunnel: w240 -> [w294]
      tunnel: [w292] -> w239 mode=indexing
      i -> [w295]
      n142 = case shown="Default" w295 {
        tunnel: w296 -> [w298 w304 _]
        tunnel: w294 -> [w299 _ _]
        tunnel: w293 -> [_ w303 _]
        tunnel: [w297 w302 i16 0 ("运行间隔")] -> w292
        frame 2, 3, 5..7, 10, 11, 14 {
          # "多参数"
          n143 = case shown="True" w298 {
            tunnel: w299 -> [_ w301]
            tunnel: [i16 0 ("运行间隔") w301] -> w297
            frame False {
            }
            frame True {
            }
          }
        }
        frame 0, 1, 4, 8, 9 {
          # "湿化学"
          n144 = case shown="True" w304 {
            tunnel: w303 -> [_ w306]
            tunnel: [i16 0 ("运行间隔") w306] -> w302
            frame False {
            }
            frame True {
            }
          }
        }
        frame Default {
        }
      }
    }
    n145 = local write "写入仪器告警信息"(w185) -> ()
    n146 = local write "写入试剂余量"(w269) -> ()
    n147 = Insert Into Array(array=u16[] [] ("values to write"), index=0 ("索引"), new element #1=w285, new element #2=w275, new element #3=w277, new element #4=w279, new element #5=w281, new element #6=w283, new element #7=w286, new element #8=w288, new element #9=w238, new element #10=w237, new element #11=w236, new element #12=w235, new element #13=w234, new element #14=w215, new element #15=w213, new element #16=w211, new element #17=w209, new element #18=w207, new element #19=w192) -> (w273:u16[])
    n148 = local write "写入系统仪器状态"(w273) -> ()
    n149 = Type Cast(type=u16[] [], x=w155) -> (*(type *) &x=w148:u16[])
    n150 = Index Array(array=w181) -> (element=w182:path)  [unwired: 1 in]
    n151 = local write "写入关键参数"(w222) -> ()
    n152 = local write "写入校准点信息"(w205) -> ()
    n153 = call <vilib>:"FileVersionInfo.vi"("Application Path in"=w182) -> ("File Version Info"=w177:string)  [unwired: 7 in, 3 out]
    n154 = Increment(x=w156) -> (x+1=w149:u16)
    n155 = Array Subset(array=w148, length=6 ("长度")) -> (w146:u16[])  [unwired: 1 in]
    n156 = Greater Or Equal?(x=w149, y=u16 5) -> (x >= y?=w153:bool)
    n157 = Insert Into Array(array=u16[] [] ("values to write"), index=0 ("索引"), new element #1=w149, new element #2=w146) -> (w150:u16[])
    n158 = Select(t=u16 0 ("y"), s=w153, f=w149) -> (s? t:f=w152:u16)
    n159 = local write "写入仪器固件"(w150) -> ()
    n160 = Concatenate Strings("V" ("字符串"), w177) -> (w179:string)
    n161 = Type Cast(type=u16[] [], x=w179) -> (*(type *) &x=w176:u16[])
    n162 = local write "写入系统版本信息"(w176) -> ()
    n163 = Insert Into Array(array=u16[] [] ("values to write"), index=0 ("索引"), new element=w239) -> (w252:u16[])
    n164 = local write "写入各参数测量间隔"(w252) -> ()
  }
  n165 = while {
    shift-right: [w356] -> _
    shift-left: _ -> [w358]
    shift-right: [w353] -> _
    shift-left: _ -> [w355]
    shift-right: [w314] -> _
    shift-left: u16[] [0, 0, 0, 0, 0, 0, 0, 0, 0, 0, 0, 0, 0, 0, 0, 0, 0, 0, 0, 0] ("初始化的数组") -> [w313]
    stop <- FALSE stop-if-true
    # "read"
    n166 = Wait (ms)(milliseconds to wait=u32 200 ("等待时间（毫秒）")) -> ()  [unwired: 1 out]
    n167 = local read "读取采水泵阀"() -> (w316:u16[])
    n168 = local read "读取反控命令"() -> (w348:u16[])
    n169 = Array Subset(array=w316, length=20 ("长度")) -> (w314:u16[])  [unwired: 1 in]
    n170 = Index Array(array=w348, index #2=14 ("索引")) -> (element #1=w356:u16, element #2=w353:u16, element #3=w320:u16, element #4=w319:u16)  [unwired: 3 in]
    n171 = Index Array(array=w348, index #3=2 ("索引"), index #4=3 ("索引"), index #5=8 ("索引"), index #6=10 ("索引"), index #8=30 ("索引")) -> (element #3=w347:u16, element #4=w346:u16, element #5=w334:u16, element #6=w343:u16, element #8=w342:u16, element #9=w341:u16, element #10=w340:u16, element #11=w339:u16, element #12=w338:u16, element #13=w337:u16, element #14=w336:u16, element #15=w331:u16, element #16=w310:u16, element #17=w308:u16)  [unwired: 12 in, 3 out]
    n172 = call "反控启动.vi"("启动参数"=w342, "启动类型"=启动命令类型."标样核查") -> ()  [unwired: 9 in, 1 out]
    n173 = call "反控启动.vi"("启动参数"=w339, "启动类型"=启动命令类型."零点核查") -> ()  [unwired: 9 in, 1 out]
    n174 = call "反控启动.vi"("启动参数"=w347, "启动类型"=启动命令类型."启动整机") -> ()  [unwired: 9 in, 1 out]
    n175 = call "反控启动.vi"("启动参数"=w340, "启动类型"=启动命令类型."平行样测试") -> ()  [unwired: 9 in, 1 out]
    n176 = call "反控启动.vi"("启动参数"=w334, "启动类型"=启动命令类型."启动系统全面清洗") -> ()  [unwired: 9 in, 1 out]
    n177 = call "反控启动.vi"("启动参数"=w346, "启动类型"=启动命令类型."停止整机") -> ()  [unwired: 9 in, 1 out]
    n178 = call "反控启动.vi"("启动参数"=w338, "启动类型"=启动命令类型."跨度核查") -> ()  [unwired: 9 in, 1 out]
    n179 = call "反控启动.vi"("启动参数"=w331, "启动类型"=启动命令类型."水样测试") -> ()  [unwired: 9 in, 1 out]
    n180 = Not Equal?(x=w356, y=w358) -> (x != y?=w357:bool)
    n181 = Not Equal?(x=w353, y=w355) -> (x != y?=w354:bool)
    n182 = Build Array(w320, w319) -> (w318:u16[])
    n183 = call <vilib>:"Value Has Changed PtByPt.vi"("input data point"=w343) -> ("has changed"=w345:bool, "output data point"=w344:dbl)  [unwired: 1 in]
    n184 = for {
      tunnel: w314 -> [w364] mode=indexing
      tunnel: w313 -> [w366] mode=indexing
      tunnel: u16 876 ("starting address") -> [w363]
      i -> [w362]
      n185 = Not Equal?(x=w364, y=w366) -> (x != y?=w365:bool)
      n186 = case shown="True" w365 {
        tunnel: w362 -> [_ w373]
        tunnel: w364 -> [_ w368]
        tunnel: w363 -> [_ w371]
        tunnel: w362 -> [_ w370]
        frame False {
        }
        frame True {
          # "变更"
          n187 = Add(x=w371, y=w370) -> (x+y=w369:i32)
          n188 = In Range and Coerce(upper limit=9 ("上限"), x=w373, lower limit=0 ("下限")) -> (In Range?=w375:bool)  [unwired: 1 out]
          n189 = case shown="False" w375 {
            tunnel: w368 -> [w393 w404]
            tunnel: [w392 w403] -> w374
            tunnel: w373 -> [w391 w402]
            tunnel: [w389 w401] -> w372
            tunnel: [w388 w400] -> w367
            frame False {
              # "阀"
              n190 = case shown="2" w393 {
                tunnel: [enum16{"清洗", "开泵X", "开阀X", "关泵X", "关阀X"}."关阀X" ("测试模式") enum16{"清洗", "开泵X", "开阀X", "关泵X", "关阀X"}."开阀X" ("测试模式") enum16{"清洗", "开泵X", "开阀X", "关泵X", "关阀X"}."关阀X" ("测试模式")] -> w392
                tunnel: [FALSE TRUE TRUE] -> w388
                frame 0, Default {
                }
                frame 1 {
                }
                frame 2 {
                }
              }
              n191 = Subtract(x=w391, y=9) -> (x-y=w389:i32)
            }
            frame True {
              # "泵"
              n192 = case shown="2" w404 {
                tunnel: [enum16{"清洗", "开泵X", "开阀X", "关泵X", "关阀X"}."关泵X" ("测试模式") enum16{"清洗", "开泵X", "开阀X", "关泵X", "关阀X"}."开泵X" ("测试模式") enum16{"清洗", "开泵X", "开阀X", "关泵X", "关阀X"}."关泵X" ("测试模式")] -> w403
                tunnel: [FALSE TRUE TRUE] -> w400
                frame 0, Default {
                }
                frame 1 {
                }
                frame 2 {
                }
              }
              n193 = Increment(x=w402) -> (x+1=w401:i32)
            }
          }
          n194 = case shown="True" w367 {
            tunnel: w374 -> [_ w385]
            tunnel: w372 -> [_ w383]
            tunnel: w369 -> [_ w381]
            frame False {
            }
            frame True {
              n195 = Bundle By Name(cluster=T24 {"测试模式"=enum."开泵X", "值"=0} ("测试模式"), "测试模式"=w385, "值"=w383) -> (w384:T24)
              n196 = call "反控启动.vi"("测试模式"=w384, "启动类型"=启动命令类型."启动采水泵阀") -> ("error out"=w382:errorcluster)  [unwired: 9 in]
              n197 = local read "MB引用"() -> (w378:refnum<class "Modbus Slave.lvclass">)
              n198 = call-dynamic "Write Single Holding Register.vi"("error in"=w382, "register to write"=u16 0, "address"=w381, "Modbus slave in"=w378) -> ("error out"=w379:errorcluster)  [unwired: 6 in, 1 out]
              n199 = call <vilib>:"Clear Errors.vi"("error in (no error)"=w379) -> ()  [unwired: 5 in, 2 out]
            }
          }
        }
      }
    }
    n200 = case shown="True" w345 {
      tunnel: w344 -> [_ w411]
      frame False {
      }
      frame True {
        # "值改变"
        n201 = case shown="1" w411 {
          frame 0, Default {
          }
          frame 1 {
            w416 = "超标留样启动交互" ("名称（未命名）")
            n202 = Obtain Queue(name (unnamed)=w416, element data type=w416) -> (queue out=w412:refnum<queue>, error out=w413:errorcluster)  [unwired: 3 in, 1 out]
            n203 = call "执行结果反馈与日志存储.vi"("日志信息"="【超标留样启动】", "error out"=T5 {"status"=FALSE, "代码"=1, "source"=""}, "设备"="超标留样") -> ()  [unwired: 9 in]
            n204 = Enqueue Element(queue=w412, element="启动留样" ("名称（未命名）"), error in (no error)=w413) -> (queue out=w414:refnum<queue>, error out=w415:errorcluster)  [unwired: 1 in, 1 out]
            n205 = Release Queue(queue=w414, error in (no error)=w415) -> ()  [unwired: 1 in, 3 out]
          }
        }
      }
    }
    n206 = call "反控启动.vi"("启动参数"=w337, "启动类型"=启动命令类型."校零") -> ()  [unwired: 9 in, 1 out]
    n207 = case shown="True" w357 {
      tunnel: w356 -> [_ w428]
      frame False {
      }
      frame True {
        # "值改变"
        n208 = flat-sequence {
          tunnel: w428 -> [w429]
          frame #0 {
            n209 = global read "modbus slave全局.vi" "与系统交互"() -> (w431:T6)
            n210 = Bundle By Name(cluster=w431, "运行模式"=w429) -> (w430:T6)
            n211 = call "系统 interface write.vi"("与系统交互"=w430) -> ()  [unwired: 11 in]
          }
          frame #1 {
            n212 = call "执行结果反馈与日志存储.vi"("日志信息"="变更【运行模式】", "error out"=T5 {"status"=FALSE, "代码"=1, "source"=""}, "设备"="系统") -> ()  [unwired: 9 in]
          }
        }
      }
    }
    n213 = call "HexToFloat.vi"("数组"=w318) -> ("FLOAT"=w321:sgl[])  [unwired: 10 in]
    n214 = case shown="True" w354 {
      tunnel: w353 -> [_ w421]
      frame False {
      }
      frame True {
        # "值改变"
        n215 = flat-sequence {
          tunnel: w421 -> [w422]
          frame #0 {
            n216 = global read "modbus slave全局.vi" "与系统交互"() -> (w424:T6)
            n217 = Bundle By Name(cluster=w424, "运行间隔"=w422, "多参数运行间隔"=w422) -> (w423:T6)
            n218 = call "系统 interface write.vi"("与系统交互"=w423) -> ()  [unwired: 11 in]
          }
          frame #1 {
            n219 = call "执行结果反馈与日志存储.vi"("日志信息"="变更【运行间隔】", "error out"=T5 {"status"=FALSE, "代码"=1, "source"=""}, "设备"="系统") -> ()  [unwired: 9 in]
          }
        }
      }
    }
    n220 = call "反控启动.vi"("启动参数"=w336, "启动类型"=启动命令类型."校标") -> ()  [unwired: 9 in, 1 out]
    n221 = Index Array(array=w321) -> (element=w317:sgl)  [unwired: 1 in]
    n222 = call "反控启动.vi"("加标体积"=w317, "启动参数"=w341, "启动类型"=启动命令类型."加标回收") -> ()  [unwired: 8 in, 1 out]
    n223 = call "反控启动.vi"("启动参数"=w310, "启动类型"=启动命令类型."仪表校准") -> ()  [unwired: 9 in, 1 out]
    n224 = call "反控启动.vi"("启动参数"=w308, "启动类型"=启动命令类型."仪表重启") -> ()  [unwired: 9 in, 1 out]
  }
  n225 = Obtain Queue(name (unnamed)="对接平台反控" ("名称（未命名）"), element data type=cluster{"命令":string} {"命令"=""}) -> (queue out=w7:refnum<queue>, error out=w6:errorcluster)  [unwired: 3 in, 1 out]
  n226 = Enqueue Element(queue=w7, element=cluster{"命令":string} {"命令"="open"} ("元素"), error in (no error)=w6) -> (queue out=w4:refnum<queue>, error out=w3:errorcluster)  [unwired: 1 in, 1 out]
  n227 = while {
    tunnel: w4 -> [w442]
    tunnel: w3 -> [w440]
    stop <- FALSE stop-if-true
    # "入队列"
    n228 = Get Queue Status(queue=w442, error in (no error)=w440) -> (queue out=w441:refnum<queue>, error out=w439:errorcluster, # elements in queue=w438:i32)  [unwired: 1 in, 5 out]
    n229 = Wait (ms)(milliseconds to wait=u32 200 ("等待时间（毫秒）")) -> ()  [unwired: 1 out]
    n230 = Equal To 0?(x=w438) -> (x = 0?=w437:bool)
    n231 = case shown="True" w437 {
      tunnel: w441 -> [_ w451]
      tunnel: w439 -> [_ w450]
      frame False {
      }
      frame True {
        w446 = cluster{"命令":string} {"命令"=""} ("元素")
        n232 = Bundle By Name(cluster=w446, "命令"="读取") -> (w443:cluster{"命令":string})
        n233 = Bundle By Name(cluster=w446, "命令"="写入") -> (w445:cluster{"命令":string})
        n234 = Enqueue Element(queue=w451, element=w445, error in (no error)=w450) -> (queue out=w449:refnum<queue>, error out=w448:errorcluster)  [unwired: 1 in, 1 out]
        n235 = Enqueue Element(queue=w449, element=w443, error in (no error)=w448) -> ()  [unwired: 1 in, 3 out]
      }
    }
  }
  n236 = while {
    tunnel: w4 -> [w470]
    tunnel: w3 -> [w469]
    shift-right: [w459] -> _
    shift-left: _ -> [w466]
    shift-right: [w455] -> _
    shift-left: _ -> [w465]
    stop <- FALSE stop-if-true
    # "main"
    n237 = Dequeue Element(queue=w470, error in (no error)=w469) -> (queue out=w457:refnum<queue>, element=w468:cluster{"命令":string})  [unwired: 1 in, 2 out]
    n238 = Unbundle By Name(w468) -> ("命令"=w467:string)
    n239 = case shown="\"读取\", Default" w467 {
      tunnel: [w483 w486 w491 w566 w613] -> w460
      tunnel: [w484 w487 w490 w565 w612] -> w461
      tunnel: w466 -> [w482 w486 w538 w610 w615]
      tunnel: w465 -> [w481 w488 w537 w609 w614]
      frame "open" {
        n240 = call-dynamic "Shutdown.vi"("error in"=w481, "Modbus slave in"=w482) -> ("error out"=w480:errorcluster)  [unwired: 9 in]
        n241 = call <vilib>:"Clear Errors.vi"("error in (no error)"=w480) -> ("error out"=w479:errorcluster)  [unwired: 5 in, 1 out]
        n242 = call-poly <vilib>:"Create Modbus Instance.vi"("error in"=w479, "port (502)"=u16 502) -> ("error out"=w484:errorcluster, "TCP slave instance"=w483:refnum<class "Modbus Slave.lvclass">)  [unwired: 8 in]
      }
      frame "close" {
        n243 = call-dynamic "Shutdown.vi"("error in"=w488, "Modbus slave in"=w486) -> ("error out"=w487:errorcluster)  [unwired: 9 in]
      }
      frame "读取", Default {
        n244 = call-dynamic "Read Holding Registers.vi"("error in"=w537, "number of inputs"=u16 40, "starting address"=u16 0, "Modbus slave in"=w538) -> ("error out"=w529:errorcluster, "register values"=w534:u16[], "Modbus slave out"=w530:refnum<class "Modbus Slave.lvclass">)  [unwired: 5 in]
        n245 = case shown="No Error" w529 {
          tunnel: w534 -> [w564 _]
          frame No Error {
            "读取反控命令" <- w564
          }
          frame Error {
          }
        }
        n246 = call-dynamic "Read Holding Registers.vi"("error in"=w529, "number of inputs"=u16 256, "starting address"=u16 256, "Modbus slave in"=w530) -> ("error out"=w524:errorcluster, "register values"=w533:u16[], "Modbus slave out"=w525:refnum<class "Modbus Slave.lvclass">)  [unwired: 5 in]
        n247 = case shown="No Error" w524 {
          tunnel: w533 -> [w563 _]
          frame No Error {
            "读取关键参数" <- w563
          }
          frame Error {
          }
        }
        n248 = call-dynamic "Read Holding Registers.vi"("error in"=w524, "number of inputs"=u16 22, "starting address"=u16 1000, "Modbus slave in"=w525) -> ("error out"=w519:errorcluster, "register values"=w526:u16[], "Modbus slave out"=w521:refnum<class "Modbus Slave.lvclass">)  [unwired: 5 in]
        n249 = case shown="No Error" w519 {
          tunnel: w526 -> [w562 _]
          frame No Error {
            "读取各参数测量间隔" <- w562
          }
          frame Error {
          }
        }
        n250 = call-dynamic "Read Holding Registers.vi"("error in"=w519, "number of inputs"=u16 1, "starting address"=u16 858, "Modbus slave in"=w521) -> ("error out"=w510:errorcluster, "register values"=w520:u16[], "Modbus slave out"=w509:refnum<class "Modbus Slave.lvclass">)  [unwired: 5 in]
        n251 = Index Array(array=w520) -> (element=w518:u16)  [unwired: 1 in]
        n252 = call-dynamic "Read Holding Registers.vi"("error in"=w510, "number of inputs"=u16 1, "starting address"=u16 866, "Modbus slave in"=w509) -> ("error out"=w502:errorcluster, "register values"=w513:u16[], "Modbus slave out"=w503:refnum<class "Modbus Slave.lvclass">)  [unwired: 5 in]
        n253 = Not Equal To 0?(x=w518) -> (x != 0?=w517:bool)
        n254 = call <vilib>:"Boolean Crossing PtByPt.vi"("direction"=enum16{"either", "false-true", "true-false"}."false-true", "input"=w517) -> ("crossing"=w516:bool)  [unwired: 1 in]
        n255 = Index Array(array=w513) -> (element=w507:u16)  [unwired: 1 in]
        n256 = Not Equal To 0?(x=w507) -> (x != 0?=w508:bool)
        n257 = call-dynamic "Read Holding Registers.vi"("error in"=w502, "number of inputs"=u16 8, "starting address"=u16 868, "Modbus slave in"=w503) -> ("error out"=w493:errorcluster, "register values"=w501:u16[], "Modbus slave out"=w492:refnum<class "Modbus Slave.lvclass">)  [unwired: 5 in]
        n258 = case shown="No Error" w493 {
          tunnel: w501 -> [w540 _]
          frame No Error {
            "读取数采仪软件版本" <- w540
          }
          frame Error {
          }
        }
        n259 = call <vilib>:"Boolean Crossing PtByPt.vi"("direction"=enum16{"either", "false-true", "true-false"}."false-true", "input"=w508) -> ("crossing"=w506:bool)  [unwired: 1 in]
        n260 = call "HexToString.vi"("字符个数"=8, "数组"=w501) -> ("STRING"=w499:string[])  [unwired: 9 in]
        n261 = call-dynamic "Read Holding Registers.vi"("error in"=w493, "number of inputs"=u16 20, "starting address"=u16 876, "Modbus slave in"=w492) -> ("error out"=w490:errorcluster, "register values"=w489:u16[], "Modbus slave out"=w491:refnum<class "Modbus Slave.lvclass">)  [unwired: 5 in]
        n262 = case shown="No Error" w490 {
          tunnel: w489 -> [w539 _]
          frame No Error {
            "读取采水泵阀" <- w539
          }
          frame Error {
          }
        }
        n263 = case shown="True" w516 {
          frame False {
          }
          frame True {
            n264 = global read "modbus slave全局.vi" "与系统交互"() -> (w556:T6)
            n265 = call "系统 interface write.vi"("与系统交互"=w556) -> ()  [unwired: 11 in]
            n266 = Get Date/Time In Seconds() -> (seconds since 1Jan1904=w559:timestamp)
            n267 = Bundle By Name(cluster=T25 {"时间标识"=timestamp(0 s since 1904-01-01), "设备"="", "日志信息"="", "流程参数"=""} ("data in"), "时间标识"=w559, "设备"="平台反控", "日志信息"="工控机软件升级") -> (w558:T25)
            n268 = call "日志存储 (子VI).vi"("data in"=w558) -> ()  [unwired: 11 in]
          }
        }
        n269 = global read "modbus slave全局.vi" "与系统交互"() -> (w497:T6)
        n270 = Index Array(array=w499) -> (element=w498:string)  [unwired: 1 in]
        n271 = case shown="True" w506 {
          tunnel: w507 -> [_ w542]
          frame False {
          }
          frame True {
            n272 = case shown="1" w542 {
              tunnel: [_ "CODMn" "氨氮" "总磷" "总氮" "CODCr"] -> w546
              frame 0, Default {
              }
              frame 1 {
              }
              frame 2 {
              }
              frame 3 {
              }
              frame 4 {
              }
              frame 5 {
              }
            }
            n273 = global read "modbus slave全局.vi" "与系统交互"() -> (w543:T6)
            n274 = Bundle By Name(cluster=w543, "固件升级"=w542) -> (w541:T6)
            n275 = global write "modbus slave全局.vi" "与系统交互"(w541) -> ()
            n276 = call "系统 interface write.vi"("与系统交互"=w541) -> ()  [unwired: 11 in]
            n277 = Concatenate Strings(w546, "固件升级" ("日志信息")) -> (w544:string)
            n278 = Get Date/Time In Seconds() -> (seconds since 1Jan1904=w549:timestamp)
            n279 = Bundle By Name(cluster=T25 {"时间标识"=timestamp(0 s since 1904-01-01), "设备"="", "日志信息"="", "流程参数"=""} ("data in"), "时间标识"=w549, "设备"="平台反控", "日志信息"=w544) -> (w548:T25)
            n280 = call "日志存储 (子VI).vi"("data in"=w548) -> ()  [unwired: 11 in]
          }
        }
        n281 = Bundle By Name(cluster=w497, "软件升级"=w517, "数采仪软件版本"=w498) -> (w496:T6)
        n282 = global write "modbus slave全局.vi" "与系统交互"(w496) -> ()
      }
      frame "写入" {
        n283 = call-dynamic "Write Multiple Holding Registers.vi"("error in"=w609, "registers to write"="写入系统仪器状态", "starting address"=u16 100, "Modbus slave in"=w610) -> ("error out"=w589:errorcluster, "Modbus slave out"=w591:refnum<class "Modbus Slave.lvclass">)  [unwired: 6 in]
        n284 = call-dynamic "Write Multiple Holding Registers.vi"("error in"=w589, "registers to write"="写入采配水关键参数", "starting address"=u16 557, "Modbus slave in"=w591) -> ("error out"=w586:errorcluster, "Modbus slave out"=w587:refnum<class "Modbus Slave.lvclass">)  [unwired: 6 in]
        n285 = call-dynamic "Write Multiple Holding Registers.vi"("error in"=w586, "registers to write"="写入仪器告警信息", "starting address"=u16 768, "Modbus slave in"=w587) -> ("error out"=w582:errorcluster, "Modbus slave out"=w583:refnum<class "Modbus Slave.lvclass">)  [unwired: 6 in]
        n286 = call-dynamic "Write Multiple Holding Registers.vi"("error in"=w582, "registers to write"="写入系统版本信息", "starting address"=u16 848, "Modbus slave in"=w583) -> ("error out"=w577:errorcluster, "Modbus slave out"=w579:refnum<class "Modbus Slave.lvclass">)  [unwired: 6 in]
        n287 = call-dynamic "Write Multiple Holding Registers.vi"("error in"=w577, "registers to write"="写入系统信息", "starting address"=u16 854, "Modbus slave in"=w579) -> ("error out"=w576:errorcluster, "Modbus slave out"=w575:refnum<class "Modbus Slave.lvclass">)  [unwired: 6 in]
        n288 = call-dynamic "Write Multiple Holding Registers.vi"("error in"=w576, "registers to write"="写入关键参数", "starting address"=u16 500, "Modbus slave in"=w575) -> ("error out"=w599:errorcluster, "Modbus slave out"=w600:refnum<class "Modbus Slave.lvclass">)  [unwired: 6 in]
        n289 = call-dynamic "Write Multiple Holding Registers.vi"("error in"=w599, "registers to write"="写入试剂余量", "starting address"=u16 4000, "Modbus slave in"=w600) -> ("error out"=w603:errorcluster, "Modbus slave out"=w604:refnum<class "Modbus Slave.lvclass">)  [unwired: 6 in]
        n290 = call-dynamic "Write Multiple Holding Registers.vi"("error in"=w603, "registers to write"="写入各参数测量间隔", "starting address"=u16 1200, "Modbus slave in"=w604) -> ("error out"=w594:errorcluster, "Modbus slave out"=w595:refnum<class "Modbus Slave.lvclass">)  [unwired: 6 in]
        n291 = call-dynamic "Write Multiple Holding Registers.vi"("error in"=w594, "registers to write"="写入校准点信息", "starting address"=u16 1400, "Modbus slave in"=w595) -> ("error out"=w573:errorcluster, "Modbus slave out"=w574:refnum<class "Modbus Slave.lvclass">)  [unwired: 6 in]
        n292 = call-dynamic "Write Multiple Holding Registers.vi"("error in"=w573, "registers to write"="写入仪器固件", "starting address"=u16 859, "Modbus slave in"=w574) -> ("error out"=w567:errorcluster, "Modbus slave out"=w569:refnum<class "Modbus Slave.lvclass">)  [unwired: 6 in]
        n293 = call-dynamic "Write Multiple Holding Registers.vi"("error in"=w567, "registers to write"="写入数据传输软件升级", "starting address"=u16 867, "Modbus slave in"=w569) -> ("error out"=w565:errorcluster, "Modbus slave out"=w566:refnum<class "Modbus Slave.lvclass">)  [unwired: 6 in]
      }
      frame "反馈" {
        n294 = global read "modbus slave全局.vi" "执行结果反馈"() -> (w611:u16[])
        n295 = call-dynamic "Write Multiple Holding Registers.vi"("error in"=w614, "registers to write"=w611, "starting address"=u16 4608, "Modbus slave in"=w615) -> ("error out"=w612:errorcluster, "Modbus slave out"=w613:refnum<class "Modbus Slave.lvclass">)  [unwired: 6 in]
      }
    }
    n296 = property class="Modbus Slave"(reference=w460, error in=w461) -> (reference out=w459:refnum<class "Modbus Slave.lvclass">, error out=w456:errorcluster, "Data Access:Daemon Error"=w458:errorcluster, "Data Access:Daemon Status"=→"Daemon Status":T2, "Data Access:TCP Connection Count"=→"TCP Connection Count":u32, "Data Access:TCP Connection List"=→"TCP Connection List":T1[])
    "MB引用" <- w459
    n297 = Unbundle By Name(w461) -> ("status"=w463:bool)
    n298 = Not(x=w463) -> (.not. x?=→"status":bool)
    n299 = case shown="Error" w458 {
      selector: w458 -> [_ w471]
      tunnel: w457 -> [_ w473]
      tunnel: w456 -> [_ _]
      tunnel: [_ w471] -> w455
      frame No Error {
      }
      frame Error {
        n300 = flat-sequence {
          tunnel: w473 -> [w475]
          tunnel: [w475] -> w472
          tunnel: w472 -> [w478]
          frame #0 {
            n301 = Wait (ms)(milliseconds to wait=u32 1000 ("等待时间（毫秒）")) -> ()  [unwired: 1 out]
          }
          frame #1 {
            n302 = Flush Queue(queue=w478) -> (queue out=w476:refnum<queue>)  [unwired: 1 in, 2 out]
            n303 = Enqueue Element(queue=w476, element=cluster{"命令":string} {"命令"="open"} ("元素")) -> ()  [unwired: 2 in, 3 out]
          }
        }
      }
    }
  }
